vi "GT Compile.vi"(8 "error in (no error)":errorcluster caption="错误输入（无错误）", 9 "pWrongInfo":T1, 10 "pFileName":string, 11 "cardNum":i16) -> (0 "error out":errorcluster caption="错误输出", 1 "pWrongInfo out":T1, 2 "pFileName out":string, 3 "pFileName":string, 4 "function return":i16, 5 "pMessage":string)   [LabVIEW 2014, in "gts.lvlib"]
doc: "GT_API GT_Compile(short cardNum,char *pFileName,TCompileInfo *pWrongInfo);"
uses:
  <vilib>/Utility/importsl/GetValueByPointer/datatype.ctl
  <vilib>/Utility/importsl/GetValueByPointer/GetValueByPointer.xnode
  gts.lvlib
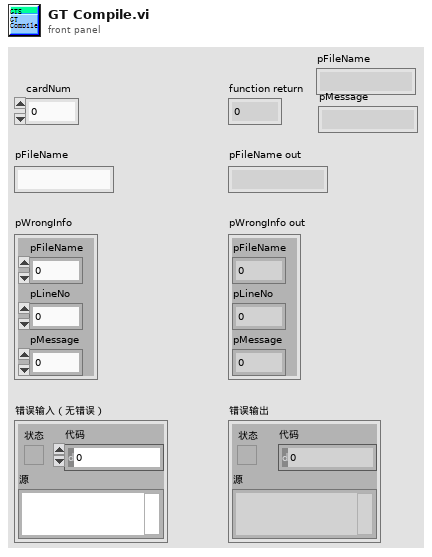
[diagram p1: front panel]
types:
  T1 = cluster{"pFileName":u32, "pLineNo":u32, "pMessage":u32}
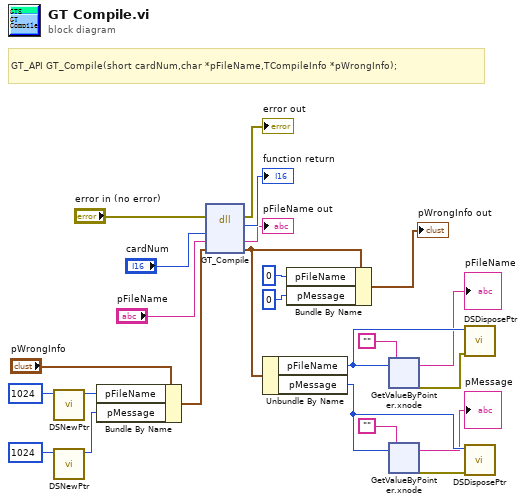
[diagram p0: block diagram]
diagram:
  # "GT_API GT_Compile(short cardNum,char *pFileName,TCompileInfo *pWrongInfo);"
  n1 = call <vilib>:"DSNewPtr.vi"("Size"=u64 1024) -> ("Pointer"=w17:u64)  [unwired: 9 in, 1 out]
  n2 = call <vilib>:"DSNewPtr.vi"("Size"=u64 1024) -> ("Pointer"=w15:u64)  [unwired: 9 in, 1 out]
  n3 = Bundle By Name(cluster="pWrongInfo", "pFileName"=w17, "pMessage"=w15) -> (w16:T1)
  n4 = dll-call lib="PTH2habs D固高科技资料GTS控制卡GTS卡18年上半年资料dllVC32bit\nmulti_cardgts.*" fn="GT_Compile"(error in="error in (no error)", "cardNum"="cardNum", "pFileName"="pFileName", "pWrongInfo"=w16) -> (error out=→"error out":errorcluster, →"function return":i16, "pFileName"=→"pFileName out":string, "pWrongInfo"=w6:T1)  [unwired: 3 in, 1 out]
  n5 = Unbundle By Name(w6) -> ("pFileName"=w13:u32, "pMessage"=w9:u32)
  n6 = Bundle By Name(cluster=w6, "pFileName"=u32 0, "pMessage"=u32 0) -> (→"pWrongInfo out":T1)
  n7 = xnode "GetValueByPointer.xnode"("Pointer"=w13, "InputType"="") -> ("Output"=→"pFileName":string, "ErrorOut"=w14:errorcluster)  [unwired: 2 in]
  n8 = xnode "GetValueByPointer.xnode"("Pointer"=w9, "InputType"="") -> ("Output"=→"pMessage":string, "ErrorOut"=w10:errorcluster)  [unwired: 2 in]
  n9 = call <vilib>:"DSDisposePtr.vi"("error in (no error)"=w14, "Pointer"=w13) -> ()  [unwired: 9 in, 1 out]
  n10 = call <vilib>:"DSDisposePtr.vi"("error in (no error)"=w10, "Pointer"=w9) -> ()  [unwired: 9 in, 1 out]
